vi "Read FileTx Notifier.vi"(8 "error in (no error)":errorcluster, 11 "FTP in":refnum<class "FTP.lvclass">) -> (0 "error out":errorcluster, 2 "FileTx Notifier":refnum<notifier>, 3 "FTP out":refnum<class "FTP.lvclass">)   [LabVIEW 2017, in "FTP_UpgradeCSMF.lvlib" / "FTP.lvclass"]
uses:
  FTP.lvclass
  controls/File Transfer Status.ctl
  FTP.lvclass/FTP.ctl
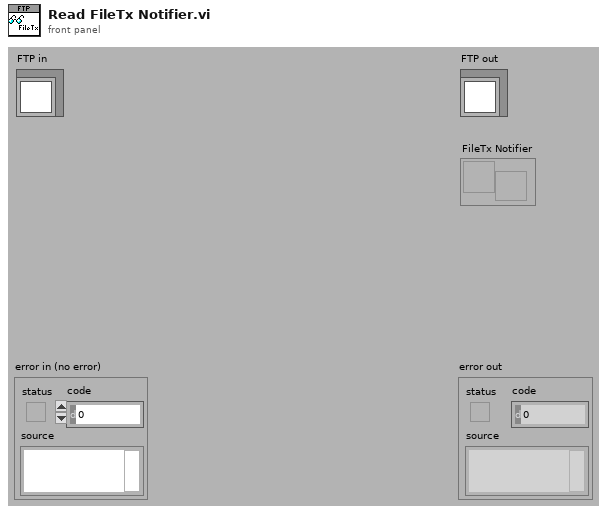
[diagram p1: front panel]
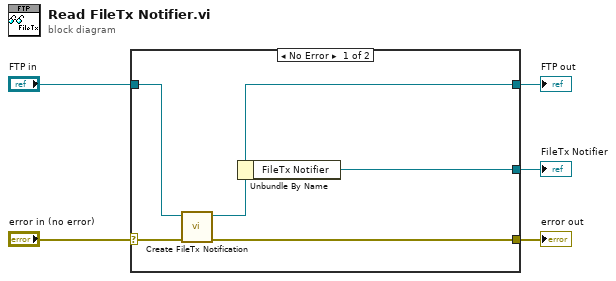
[diagram p0: block diagram]
diagram:
  n1 = case shown="No Error" "error in (no error)" {
    selector: "error in (no error)" -> [w9 w11]
    tunnel: [w6 w11] -> w4
    tunnel: [w7 w12] -> w2
    tunnel: "FTP in" -> [w8 w12]
    tunnel: [w10 _] -> w1
    frame No Error {
      n2 = call "Create FileTx Notification.vi"("error in (no error)"=w9, "FTP in"=w8) -> ("error out"=w6:errorcluster, "FTP out"=w7:refnum<class "FTP.lvclass">)  [unwired: 8 in]
      n3 = Unbundle By Name(w7) -> ("FileTx Notifier"=w10:refnum<notifier>)
    }
    frame Error {
    }
  }
  "error out" <- w4
  "FTP out" <- w2
  "FileTx Notifier" <- w1
